vi "Working12VDCChasee.vi"   [LabVIEW 2015]
uses:
  <vilib>/Aledyne-TSXperts/Arduino Compatible Compiler for LabVIEW/Code Generator/Arduino APIs/RGB LED Strip/RGB Strip Mode.ctl
  <vilib>/Aledyne-TSXperts/Arduino Compatible Compiler for LabVIEW/Code Generator/Arduino APIs/Digital/PinDirection.ctl
  <vilib>/Aledyne-TSXperts/Arduino Compatible Compiler for LabVIEW/Arduino Compatible Compiler for LabVIEW.lvlib
types:
  T1 = typedef "Arduino Compatible Compiler for LabVIEW.lvlib/PinDirection.ctl" = enum16{" INPUT", "OUTPUT", " INPUT_PULLUP"}
  T2 = typedef "Arduino Compatible Compiler for LabVIEW.lvlib/RGB Strip Mode.ctl" = u16
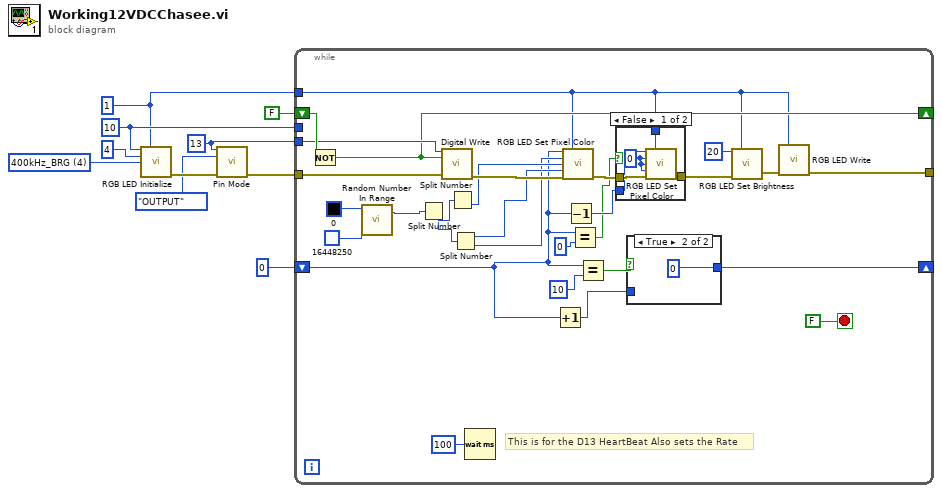
[diagram p0: block diagram]
diagram:
  w4 = u8 13 ("pin")
  w2 = u8 1 ("Instance")
  w3 = u16 10 ("Number of Pixels")
  w10 = T2 4 items=["400kHz_RGB"=0, "400kHz_GRB"=1, "400kHz_BRG"=4, "800kHz_RGB"=2, "800kHz_GRB"=3, "400kHz_BRG"=6] ("Mode")
  n1 = call <vilib>:"RGB LED Initialize.vi"("Number of Pixels"=w3, "Instance"=w2, "Pin"=u8 4, "Mode"=w10) -> ("error out"=w8:errorcluster)  [unwired: 11 in]
  n2 = call <vilib>:"Pin Mode.vi"("pin"=w4, "direction"=PinDirection."OUTPUT", "error in (no error)"=w8) -> ("error out"=w6:errorcluster)  [unwired: 12 in]
  n3 = while {
    tunnel: w6 -> [w39]
    shift-right: [w33] -> _
    shift-left: FALSE -> [w38]
    tunnel: w4 -> [w37]
    tunnel: w3 -> [_]
    tunnel: w2 -> [w18]
    tunnel: [w34] -> _
    shift-right: [w22] -> _
    shift-left: u16 0 ("Pixel") -> [w16]
    stop <- FALSE stop-if-true
    # "This is for the D13 HeartBeat Also sets the Rate"
    n4 = Not(x=w38) -> (.not. x?=w33:bool)
    n5 = call <vilib>:"Random Number In Range.vi"("max"=u32 16448250, "min"=u32 0) -> ("Random Number"=w11:u32)  [unwired: 3 in]
    n6 = Split Number(x=w11) -> (hi(x)=w31:u16, lo(x)=w30:u16)
    n7 = call <vilib>:"Digital Write.vi"("pin"=w37, "state"=w33, "error in (no error)"=w39) -> ("error out"=w36:errorcluster)  [unwired: 12 in]
    n8 = Split Number(x=w31) -> (lo(x)=w29:u8)  [unwired: 1 out]
    n9 = Split Number(x=w30) -> (hi(x)=w28:u8, lo(x)=w27:u8)
    n10 = Wait (ms)(milliseconds to wait=u32 100) -> ()  [unwired: 1 out]
    n11 = Increment(x=w16) -> (x+1=w21:u16)
    n12 = call <vilib>:"RGB LED Set Pixel Color.vi"("Pixel"=w16, "Instance"=w18, "Red"=w27, "Green"=w29, "Blue"=w28, "error in (no error)"=w36) -> ("error out"=w20:errorcluster)  [unwired: 9 in]
    n13 = Decrement(x=w16) -> (x-1=w17:u16)
    n14 = Equal?(x=w16, y=u16 0) -> (x = y?=w14:bool)
    n15 = Equal?(x=w16, y=u16 10) -> (x = y?=w23:bool)
    n16 = case shown="False" w14 {
      tunnel: w20 -> [w44 w45]
      tunnel: [w43 w45] -> w19
      tunnel: w18 -> [w42 _]
      tunnel: w17 -> [w41 _]
      frame False {
        w40 = u8 0 ("Red")
        n17 = call <vilib>:"RGB LED Set Pixel Color.vi"("Pixel"=w41, "Instance"=w42, "Red"=w40, "Green"=w40, "Blue"=w40, "error in (no error)"=w44) -> ("error out"=w43:errorcluster)  [unwired: 9 in]
      }
      frame True {
      }
    }
    n18 = case shown="True" w23 {
      tunnel: [w46 u16 0 ("Pixel")] -> w22
      tunnel: w21 -> [w46 _]
      frame False {
      }
      frame True {
      }
    }
    n19 = call <vilib>:"RGB LED Set Brightness.vi"("Brightness"=u8 20, "Instance"=w18, "error in (no error)"=w19) -> ("error out"=w35:errorcluster)  [unwired: 12 in]
    n20 = call <vilib>:"RGB LED Write.vi"("Instance"=w18, "error in (no error)"=w35) -> ("error out"=w34:errorcluster)  [unwired: 13 in]
  }
